vi "meTEC_Read_ID 105_Error Number.vi"(8 "error in (no error)":errorcluster, 9 "TEC Configuration_IN":T1={"VISA resource name"="", "Device Address"=2}, 10 "Sequence No.":u32=5552) -> (0 "error out":errorcluster, 1 "TEC Configuration_OUT":T1={"VISA resource name"="", "Device Address"=2}, 2 "Error Number (ID 105) [I32]":i32, 3 "Error Number (ID 105) [String]":string)   [LabVIEW 2019]
uses:
  TypeDefs/meTEC_Configuration.ctl
panel:
  # "--- Inputs ---"
  # "--- Outputs ---"
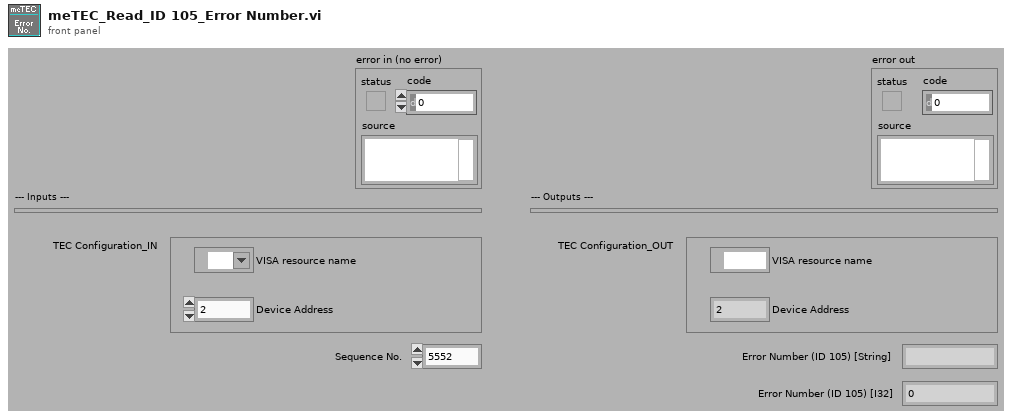
[diagram p1: front panel]
types:
  T1 = typedef "meTEC_Configuration.ctl" = cluster{"VISA resource name":refnum<visa-resource-name>, "Device Address":u16}
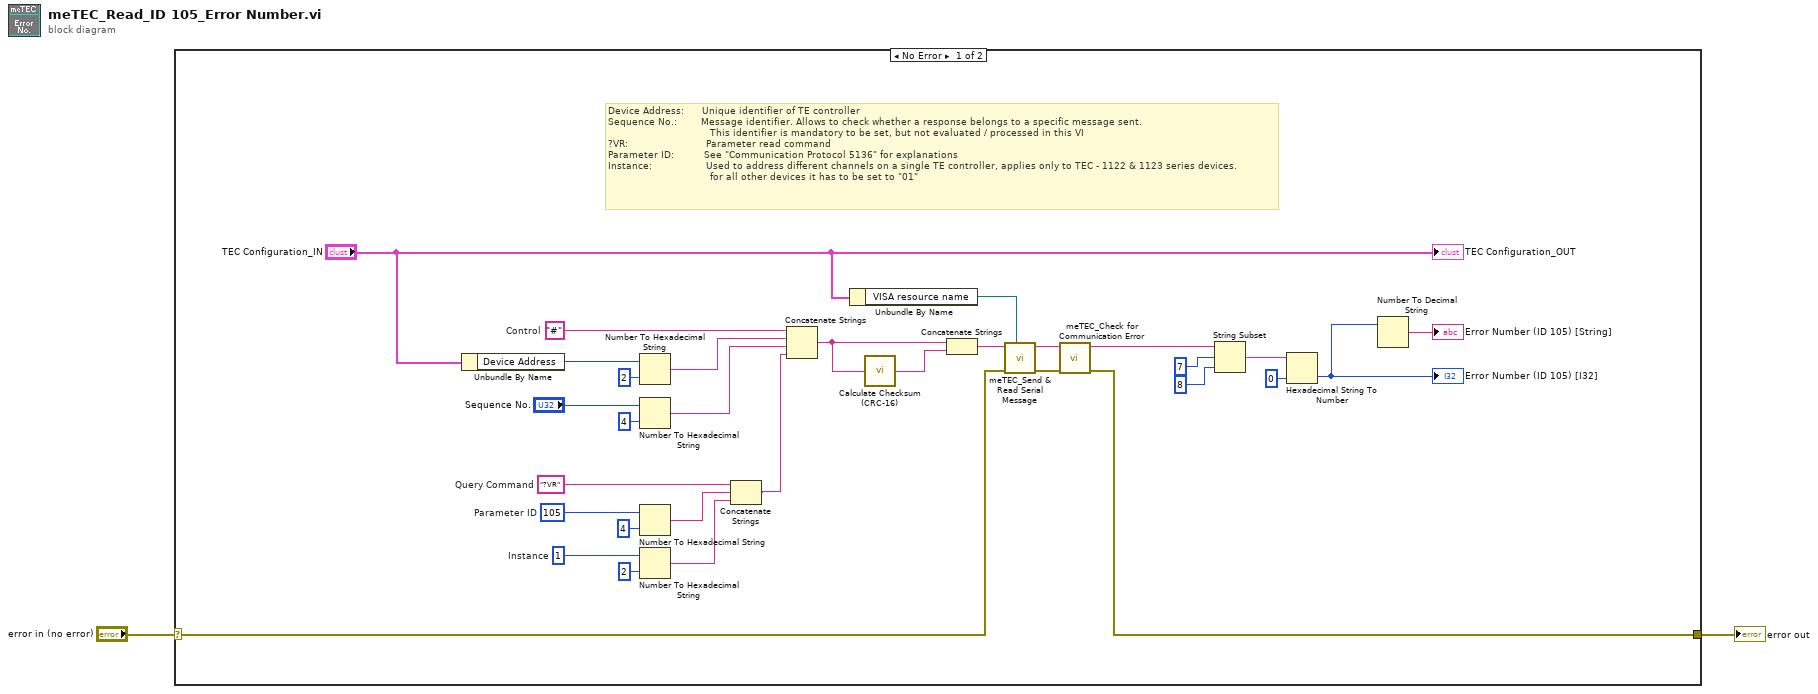
[diagram p0: block diagram]
diagram:
  n1 = case shown="No Error" "error in (no error)" {
    selector: "error in (no error)" -> [w17 w34]
    tunnel: [w5 w34] -> w2
    frame No Error {
      w6 = u8 1  # Instance
      w22 = 105  # Parameter ID
      w23 = "?VR"  # Query Command
      w31 = "#"  # Control
      # "Device Address:      Unique identifier of TE controller\nSequence No.:        Message identifier. Allows to check whether a response belongs to a specific message sent.\n                                  This identifier is mandatory to be set, but not evaluated / processed in this VI\n?VR:                          Parameter read command\nParameter ID:          See \"Communication Protocol 5136\" for explanations\nInstance:                  Used to address different channels on a single TE controller, applies only to TEC - 1122 & 1123 series devices.\n                                  for all other devices it has to be set to \"01\""
      n2 = Unbundle By Name("TEC Configuration_IN") -> ("Device Address"=w10:u16)
      n3 = Number To Hexadecimal String(1:i16 2 ("width (-)"), 2:w10) -> (0:w26:string)
      n4 = Number To Hexadecimal String(1:i16 4 ("width (-)"), 2:"Sequence No.") -> (0:w30:string)
      n5 = Number To Hexadecimal String(1:i16 4 ("width (-)"), 2:w22) -> (0:w24:string)
      n6 = Number To Hexadecimal String(1:i16 2 ("width (-)"), 2:w6) -> (0:w14:string)
      n7 = Concatenate Strings(w23, w24, w14) -> (w20:string)
      n8 = Concatenate Strings(w31, w26, w30, w20) -> (w29:string)
      n9 = Unbundle By Name("TEC Configuration_IN") -> ("VISA resource name"=w11:refnum<visa-resource-name>)
      n10 = call "Calculate Checksum (CRC-16).vi"("Message"=w29) -> ("CRC [String]"=w28:string)  [unwired: 1 in]
      n11 = Concatenate Strings(w29, w28) -> (w25:string)
      n12 = call "meTEC_Send & Read Serial Message.vi"("VISA resource name"=w11, "error in (no error)"=w17, "Serial Message"=w25) -> ("error out"=w16:errorcluster, "Serial Message_Read"=w4:string)  [unwired: 7 in]
      n13 = call "meTEC_Check for Communication Error.vi"("error in (no error)"=w16, "Serial Message_IN"=w4) -> ("error out"=w5:errorcluster, "Serial Message_OUT"=w3:string)  [unwired: 8 in]
      n14 = String Subset(string=w3, offset (0)=7, length (rest)=8 ("length (rest)")) -> (substring=w12:string)
      n15 = Hexadecimal String To Number(string=w12, default (0uL)=0 ("default (0 U32)")) -> (number=w7:i32)  [unwired: 1 in, 1 out]
      "Error Number (ID 105) [I32]" <- w7
      n16 = Number To Decimal String(number=w7) -> (decimal integer string=→"Error Number (ID 105) [String]":string)  [unwired: 1 in]
      "TEC Configuration_OUT" <- "TEC Configuration_IN"
    }
    frame Error {
    }
  }
  "error out" <- w2
